vi "Vision Processing Dashboard.vi"() -> (0 "Particle Measurements (Pixels)":dbl[][](array[numeric]))   [LabVIEW 2012]
doc: "<B>Vision Processing Dashboard</B> is a modified FRC Dashboard project that includes vision processing built into the dashboard. The dashboard takes in an image from the camera on the robot and searches for objects within the specified RGB ranges. The image and the image with the threshold are shown in the Camera Image Tab. The ranges are controlled from the Operation tab. The dashboard is set up to display the center of mass in X and Y pixels as well as the area in pixels of any objects that are located."
uses:
  <vilib>/Rock Robotics/WPI/Camera/WPI_CameraImageSize.ctl
  <vilib>/event_ctls.llb/eventvkey.ctl
  <vilib>/Utility/config.llb/Read Key (String).vi
  <vilib>/Utility/config.llb/Read Key (I32).vi
  <vilib>/Analysis/Matrix/Numeric/Conversions/Matrix To Array - RM.vi
  <vilib>/Utility/config.llb/NI_LVConfig.lvlib
  <vilib>/vision/NI_Vision_Development_Module.lvlib
  <vilib>/Analysis/Matrix/NI_Matrix.lvlib
panel:
  out "Battery Value":dbl(slide) scale=0.0..14.0 scale format="%#_2e"
  out "Battery":sgl(graph)
  out "Robot IP":string
  in  "Viewer":T1(tab)
  in  "Enable":bool
  in  "DB Camera Config":bool
  out "Image Error Message":string="Timeout in Camera Communications"
  in  "Camera Address":string="192.168.0.90"
  out "Originial":T2(plugin-control)
  out "Threshold":T2(plugin-control)
  in  "Image Size":T3=enum."320x240"
  out "Buttons 1":cluster{"1":bool, "2":bool, "3":bool}
  out "Kinect 1":cluster{"X":dbl, "Y":dbl, "Z":dbl} {"X" scale=1.0..-1.0; "Y" scale=1.0..-1.0; "Z" scale=1.0..-1.0}
  out "Buttons 2":cluster{"1":bool, "2":bool, "3":bool}
  out "Kinect 2":cluster{"X":dbl, "Y":dbl, "Z":dbl} {"X" scale=1.0..-1.0; "Y" scale=1.0..-1.0; "Z" scale=1.0..-1.0}
  out "Version":string
  out "Skeleton Picture":picture
  out "Players":i8
  out "Tree":string(tree)
  out "Mode":T4(ring)=enum."Auto Disabled"
  out "Camera IP":string
  out "JS1 Z":dbl(slide) scale=-1.0..1.0 scale format="%#_2e"
  out "JS2 Z":dbl(slide) scale=-1.0..1.0 scale format="%#_2e"
  out "Joystick 1":cluster{"X":dbl, "Y":dbl}[](graph)
  out "Joystick 2":cluster{"X":dbl, "Y":dbl}[](graph)
  out "JS Buttons 1":T5
  out "JS Buttons 2":T5
  out "MotorSlide4":dbl(slide) scale=-1.0..1.0 scale format="%#_2e"
  out "MotorSlide3":dbl(slide) scale=-1.0..1.0 scale format="%#_2e"
  out "MotorSlide2":dbl(slide) scale=-1.0..1.0 scale format="%#_2e"
  in  "MotorName3":string="Front Left"
  in  "MotorName4":string="Front Right"
  in  "MotorName1":string="Rear Left"
  in  "MotorName2":string="Rear Right"
  out "MotorChart4":dbl(graph)
  out "MotorChart3":dbl(graph)
  out "MotorChart2":dbl(graph)
  out "MotorSlide1":dbl(slide) scale=-1.0..1.0 scale format="%#_2e"
  out "MotorChart1":dbl(graph)
  in  "Dashboard Tab":enum32{"Operation", "Test", "Checklist"}(tab)
  in  "Red Range":cluster{"Lower value":dbl, "Upper Value":dbl}
  in  "Green Range":cluster{"Lower value":i32, "Upper Value":i32}
  in  "Blue Range":cluster{"Lower value":dbl, "Upper Value":dbl}
  in  "Slider":dbl(slide) scale=0.0..100.0 scale format="%#_3g"
  in  "On/Off":bool caption="Solenoid"
  in  "Test Name":u16(ring) items=["Select the test to run...", "Example Test", "-------------------------------", "List of tests is built in robot code.", "Replace with your own automated tests."]
  in  "Test Tree":string(tree)
  in  "Motor":cluster{"Value":dbl, "Enable":bool} {"Value" scale=-1.0..1.0 scale format="%#_3g"}
  out "Progress":T6 {"Test Progress" scale=0.0..100.0}
  in  "Rev/Fwd":cluster{"Forward":bool, "Reverse":bool}
  in  "Ring":u16(ring) items=["Auto", "Fixed indoor", "Fixed outdoor 1", "Fixed outdoor 2", "Fixed fluorescent 1", "Fixed fluorescent 2", "Hold current"]
  in  "Listbox":i32(listbox)
  # "Robot IP:"
  # "Drive & Motors"
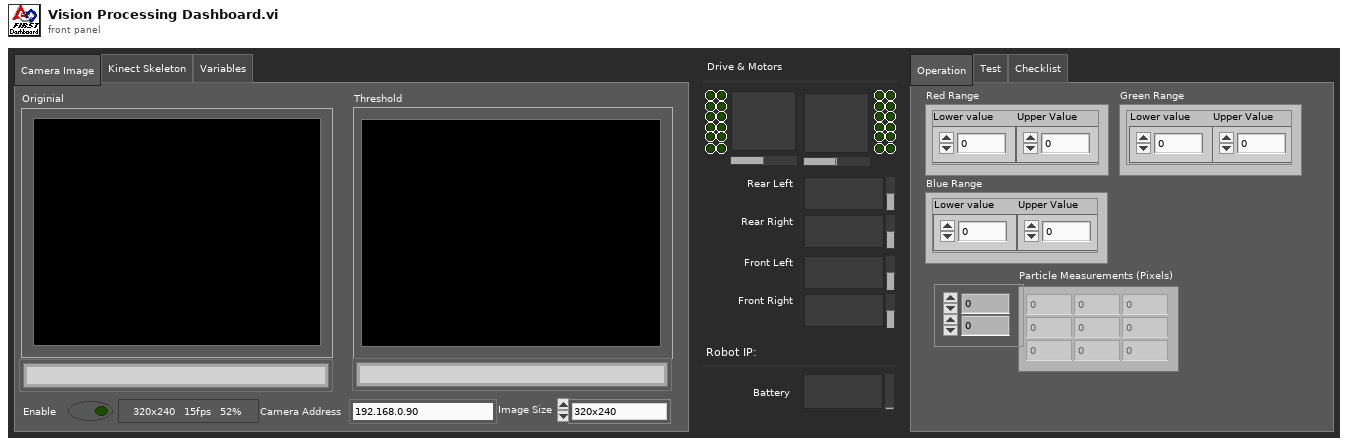
[diagram p1: front panel]
types:
  T1 = enum32{"Camera Image", "Kinect Skeleton", "Variables"}
  T2 = typedef "IMAQ Image.ctl" = refnum<image>
  T3 = typedef "WPI_CameraImageSize.ctl" = enum16{"640x480", "320x240", "160x120"}
  T4 = enum8{"Tele-Op Disabled", "Tele-Op Enabled", "Auto Disabled", "Auto Enabled", "Test Disabled", "Test Enabled", ""}
  T5 = cluster{bool, bool, bool, bool, bool, bool, bool, bool, bool, bool, bool, bool}
  T6 = cluster{"Test Progress":u8, "Test Progress Text":string}
  T7 = typedef "Image Type" = u32
  T8 = typedef "WPI_CameraDevRef.ctl" = cluster{"Camera Address":string, "CameraStatus":errorcluster, "Acquire Image Notifier":refnum<notifier>}
  T9 = typedef "LVBoundsTypeDef.ctl" = cluster{"Width":u32, "Height":u32}
  T10 = typedef "SkeletonTrackState.ctl" = enum32{"NotTracked", "PositionOnly", "Tracked"}
  T11 = cluster{"TrackingState":u8[], "Position":cluster{"x":sgl, "y":sgl, "z":sgl}, cluster{"x":sgl, "y":sgl, "z":sgl, sgl}[], "TrackState":T10}
  T12 = cluster{cluster{"ScaledToPercentRange":dbl, "ScaledToPercentRange":dbl, "ScaledToPercentRange":dbl}, cluster{bool, bool, bool}}[]
  T13 = cluster{cluster{"ScaledToPercentRange":dbl, "ScaledToPercentRange":dbl, "ScaledToPercentRange":dbl}, cluster{bool, bool, bool}}
  T14 = cluster{"ScaledToPercentRange":dbl, "ScaledToPercentRange":dbl, "ScaledToPercentRange":dbl}
  T15 = typedef "LVRectTypeDef.ctl" = cluster{"Left":i16, "Top":i16, "Right":i16, "Bottom":i16}
  T16 = typedef "Particle Parameters" = i32
  T17 = cluster{"[0]":dbl, "[1]":dbl, "[2]":dbl, "[3]":dbl, "[4]":dbl, "[5]":dbl, "[6]":dbl, "[7]":dbl, "[8]":dbl}
  T18 = cluster{"Competition mode":bool, "Robot Link":bool, "Autonomous":bool, "Enabled":bool, "E-Stop":bool, "Simulated":bool, "TestMode":bool, "Docked Window":bool}
  T19 = cluster{"Boolean Array[0]":bool, "Boolean Array[1]":bool, "Boolean Array[2]":bool, "Boolean Array[3]":bool, "Boolean Array[4]":bool, "Boolean Array[5]":bool, "Boolean Array[6]":bool, "Boolean Array[7]":bool, "Boolean Array[8]":bool, "Boolean Array[9]":bool, "Boolean Array[10]":bool, "Boolean Array[11]":bool}
  T20 = typedef "NI_LVConfig.lvlib/Config Data RefNum.ctl" = refnum<k1>
  T21 = typedef "eventvkey.ctl" = enum16{"ASCII", "Enter", "Return", "Shift", "Ctrl", "Alt", "Cmd", "Opt", "Caps", "NumLock", "Clear", "Break", "Up", "Down", "Left", "Right", "Insert", "Delete", "Home", "End", "PageUp", "PageDown", "Escape", "Help", "Pause", "ScrollLock", "F1", "F2", "F3", "F4", "F5", "F6", "F7", "F8", "F9", "F10", "F11", "F12", "F13", "F14", "F15", "F16", "F17", "F18", "F19", "F20", "F21", "F22", "F23", "F24", "Play", "VolumeUp", "VolumeDown", "Mute", "Two Byte Char"}
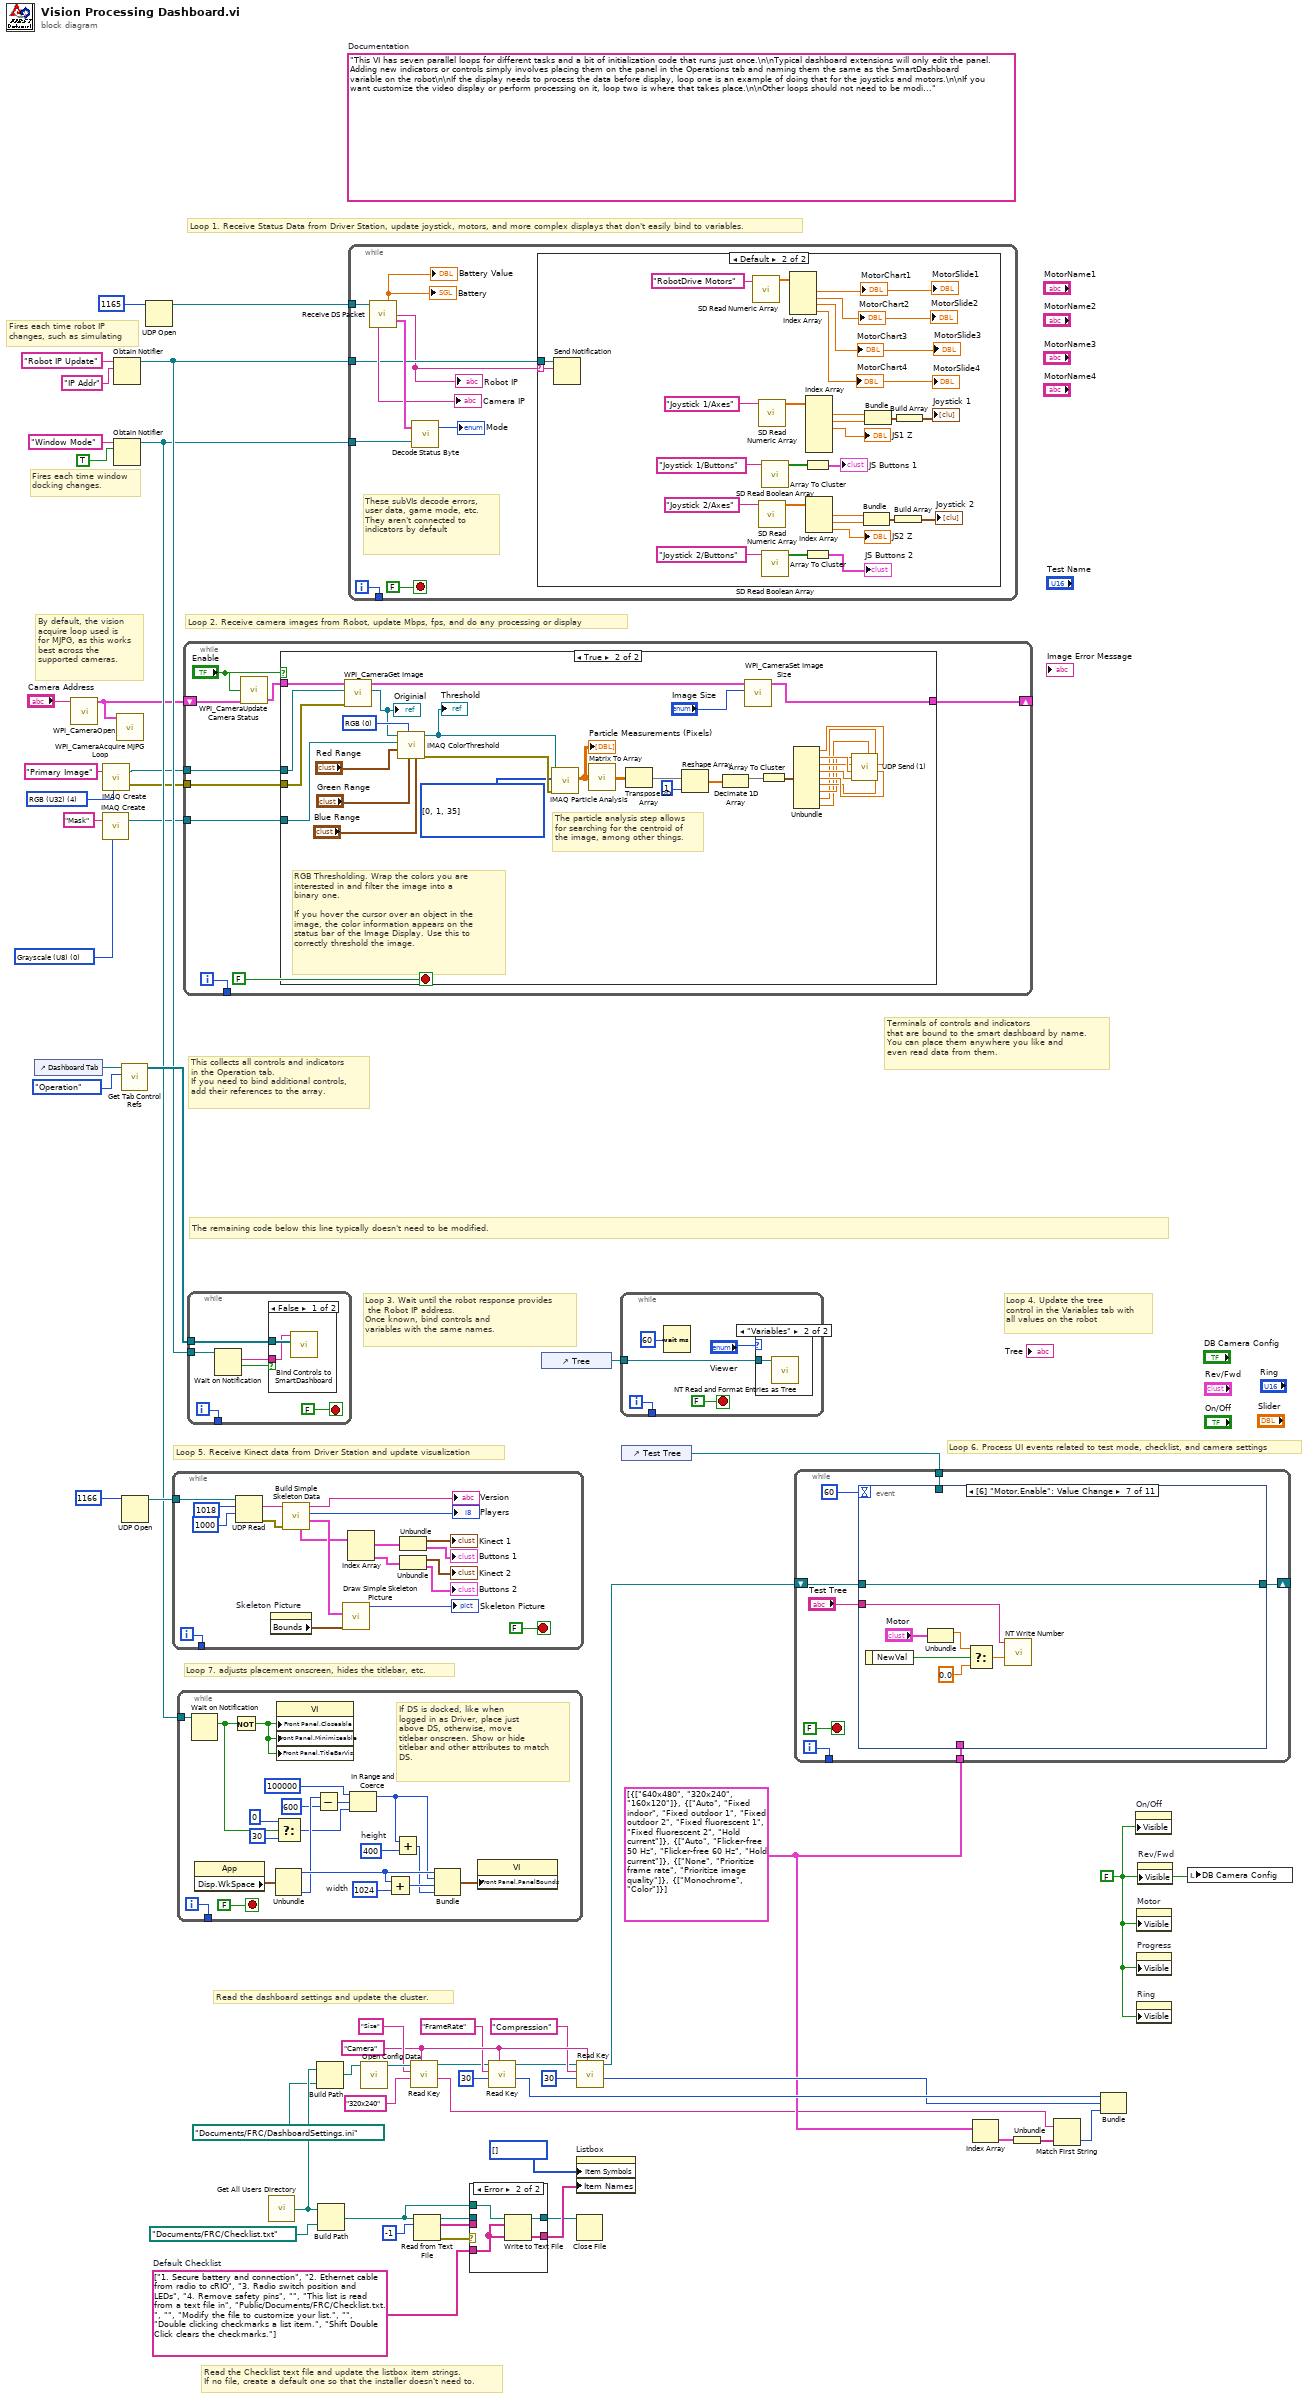
[diagram p0: block diagram]
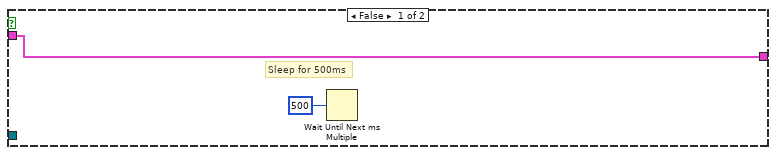
[diagram p3: hidden frame]
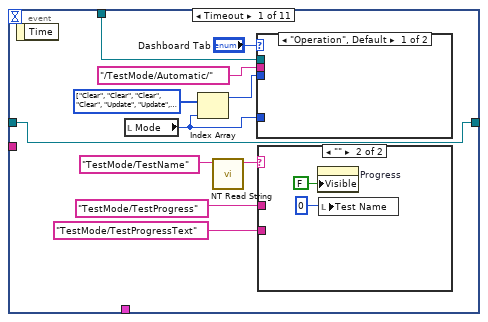
[diagram p5: hidden frame]
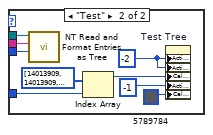
[diagram p6: hidden frame]
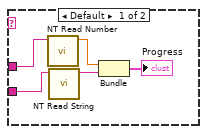
[diagram p7: hidden frame]
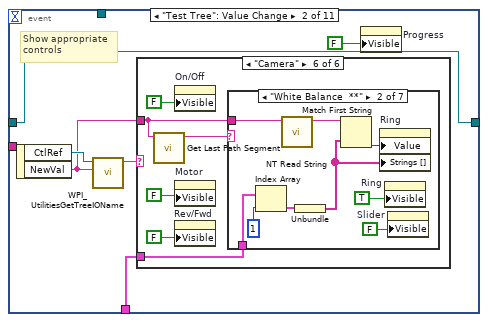
[diagram p8: hidden frame]
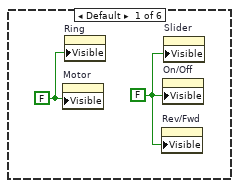
[diagram p9: hidden frame]
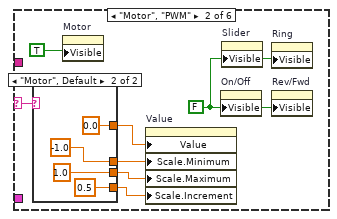
[diagram p10: hidden frame]
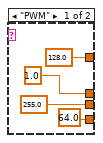
[diagram p11: hidden frame]
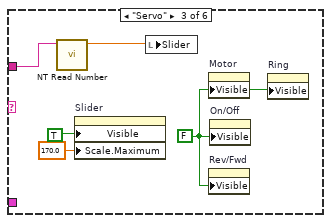
[diagram p12: hidden frame]
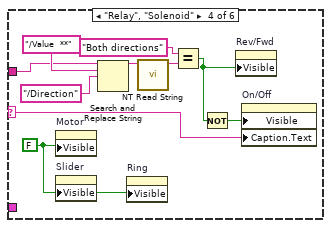
[diagram p13: hidden frame]
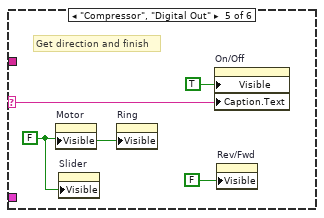
[diagram p14: hidden frame]
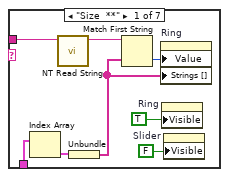
[diagram p15: hidden frame]
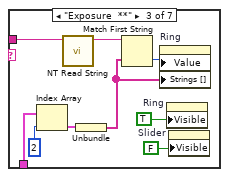
[diagram p16: hidden frame]
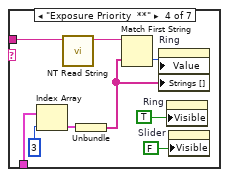
[diagram p17: hidden frame]
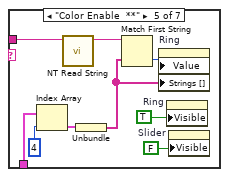
[diagram p18: hidden frame]
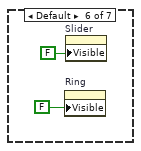
[diagram p19: hidden frame]
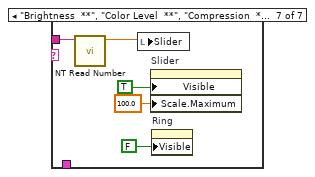
[diagram p20: hidden frame]
diagram:
  w7 = T7 0 items=["Grayscale (U8)", "Grayscale (I16)", "Grayscale (SGL)", "Complex (CSG)", "RGB (U32)", "HSL (U32)", "RGB (U64)", "Grayscale (U16)"] ("Image Type")
  w9 = T7 4 items=["Grayscale (U8)", "Grayscale (I16)", "Grayscale (SGL)", "Complex (CSG)", "RGB (U32)", "HSL (U32)", "RGB (U64)"] ("Image Type")
  w29 = "Camera"
  w21 = cluster{string[]}[] [{["640x480", "320x240", "160x120"]}, {["Auto", "Fixed indoor", "Fixed outdoor 1", "Fixed outdoor 2", "Fixed fluorescent 1", "Fixed fluorescent 2", "Hold current"]}, {["Auto", "Flicker-free 50 Hz", "Flicker-free 60 Hz", "Hold current"]}, {["None", "Prioritize frame rate", "Prioritize image quality"]}, {["Monochrome", "Color"]}]
  w37 = string[] ["1. Secure battery and connection", "2. Ethernet cable from radio to cRIO", "3. Radio switch position and LEDs", "4. Remove safety pins", "", "This list is read from a text file in", "Public/Documents/FRC/Checklist.txt.", "", "Modify the file to customize your list.", "", "Double clicking checkmarks a list item.", "Shift Double Click clears the checkmarks."]  # Default Checklist
  w35 = FALSE ("Visible")
  (unwired) "This VI has seven parallel loops for different tasks and a bit of initialization code that runs just once.\n\nTypical dashboard extensions will only edit the panel. Adding new indicators or controls simply involves placing them on the panel in the Operations tab and naming them the same as the SmartDashboard variable on the robot\n\nIf the display needs to process the data before display, loop one is an example of doing that for the joysticks and motors.\n\nIf you want customize the video display or perform processing on it, loop two is where that takes place.\n\nOther loops should not need to be modified. They are pretty standard, and document the task they perform."  # Documentation
  # "By default, the vision\nacquire loop used is\nfor MJPG, as this works\nbest across the\nsupported cameras."
  # "Fires each time robot IP\nchanges, such as simulating"
  # "Fires each time window\ndocking changes."
  # "Read the Checklist text file and update the listbox item strings.\nIf no file, create a default one so that the installer doesn't need to."
  # "This collects all controls and indicators\nin the Operation tab.\nIf you need to bind additional controls,\nadd their references to the array."
  # "The remaining code below this line typically doesn't need to be modified."
  # "Loop 6. Process UI events related to test mode, checklist, and camera settings"
  # "Read the dashboard settings and update the cluster."
  # "Terminals of controls and indicators\nthat are bound to the smart dashboard by name.\nYou can place them anywhere you like and\neven read data from them."
  # "Loop 4. Update the tree\ncontrol in the Variables tab with\nall values on the robot"
  # "Loop 3. Wait until the robot response provides\n the Robot IP address.\nOnce known, bind controls and\nvariables with the same names."
  # "Loop 5. Receive Kinect data from Driver Station and update visualization"
  # "Loop 7. adjusts placement onscreen, hides the titlebar, etc."
  # "Loop 1. Receive Status Data from Driver Station, update joystick, motors, and more complex displays that don't easily bind to variables."
  # "Loop 2. Receive camera images from Robot, update Mbps, fps, and do any processing or display"
  n1 = control-ref of="Dashboard Tab"() -> (w51:refnum<vi>)
  n2 = call <vilib>:"WPI_CameraOpen.vi"("Camera Address"="Camera Address") -> ("CameraDevRef"=w2:T8)  [unwired: 9 in, 1 out]
  n3 = call "IMAQ Create"("Image Name"="Mask", "Image Type"=w7) -> ("New Image"=w1:T2)  [unwired: 2 in, 2 out]
  n4 = call "IMAQ Create"("Image Name"="Primary Image", "Image Type"=w9) -> ("New Image"=w5:T2, "error out"=w4:errorcluster)  [unwired: 2 in, 1 out]
  n5 = Obtain Notifier(name (unnamed)="Robot IP Update", notification data type="IP Addr" ("name (unnamed)")) -> (notifier out=w48:refnum<notifier>)  [unwired: 2 in, 2 out]
  n6 = Obtain Notifier(name (unnamed)="Window Mode", notification data type=TRUE) -> (notifier out=w41:refnum<notifier>)  [unwired: 2 in, 2 out]
  n7 = call <vilib>:"WPI_CameraAcquire MJPG Loop.vi"("CameraDevRef"=w2) -> ()  [unwired: 11 in]
  n8 = call <vilib>:"Get Tab Control Refs.vi"("Page Index"=enum32{"Operation", "Test"}."Operation" ("Dashboard Tab"), "TabControl in"=w51) -> ("ControlsOnPage"=w52:refnum<vi>[])  [unwired: 9 in]
  n9 = UDP Open(11:u16 1166 ("port")) -> (port=w53:refnum<k16>)  [unwired: 2 in, 4 out]
  n10 = UDP Open(11:u16 1165 ("port")) -> (port=w55:refnum<k16>)  [unwired: 2 in, 4 out]
  n11 = while {
    tunnel: w53 -> [w73]
    tunnel: [w58] -> _
    i -> [w58]
    stop <- FALSE stop-if-true
    n12 = UDP Read(connection ID=w73, max size (548)=1018 ("bytes to read"), timeout ms (25000)=1000) -> (data out=w67:string, error out=w57:errorcluster)  [unwired: 1 in, 3 out]
    n13 = property on="Skeleton Picture" class="Pict"() -> ("Bounds"=w69:T9)  [unwired: 2 in, 2 out]
    n14 = call "Build Simple Skeleton Data.vi"("error in (no error)"=w57, "data in"=w67) -> ("Skeleton Data"=w68:T11, "NumPlayers"=→"Players":i8, "Version String"=→"Version":string, "Simple Joystick Info"=w65:T12)  [unwired: 5 in, 1 out]
    n15 = call "Draw Simple Skeleton Picture.vi"("Bounds"=w69, "Simple Skeleton"=w68) -> ("new picture out"=→"Skeleton Picture":picture)  [unwired: 9 in]
    n16 = Index Array(array=w65) -> (element #1=w64:T13, element #2=w63:T13)  [unwired: 2 in]
    n17 = Unbundle(w64) -> (→"Kinect 1":T14, →"Buttons 1":cluster{bool, bool, bool})
    n18 = Unbundle(w63) -> (→"Kinect 2":T14, →"Buttons 2":cluster{bool, bool, bool})
  }
  n19 = while {
    tunnel: w41 -> [w94]
    tunnel: [w92] -> _
    i -> [w92]
    stop <- FALSE stop-if-true
    w84 = 1024  # width
    w87 = 400  # height
    # "If DS is docked, like when\nlogged in as Driver, place just\nabove DS, otherwise, move\ntitlebar onscreen. Show or hide\ntitlebar and other attributes to match\nDS."
    n20 = Wait on Notification(notifier=w94) -> (notification=w79:bool)  [unwired: 3 in, 3 out]
    n21 = property class="App"() -> ("Disp.WkSpace"=w90:T15)  [unwired: 2 in, 2 out]
    n22 = Not(x=w79) -> (.not. x?=w93:bool)
    n23 = Unbundle(w90) -> ("Left"=w88:i16, "Bottom"=w85:i16)  [unwired: 2 out]
    n24 = Select(t=0, s=w79, f=30) -> (s? t:f=w78:i32)
    n25 = property class="VI"("Front Panel.Closeable"=w93, "Front Panel.Minimizeable"=w93, "Front Panel.TitleBarVis"=w93) -> ()  [unwired: 2 in, 2 out]
    n26 = Subtract(x=w85, y=600) -> (x-y=w82:i32)
    n27 = In Range and Coerce(upper limit=100000, x=w82, lower limit=w78) -> (coerced(x)=w76:i32)  [unwired: 1 out]
    n28 = Add(x=w88, y=w84) -> (x+y=w89:i32)
    n29 = Add(x=w76, y=w87) -> (x+y=w86:i32)
    n30 = Bundle("Left"=w88, w76, w89, w86) -> (w91:cluster{"Left":i16, i32, i32, i32})  [unwired: 1 out]
    n31 = property class="VI"("Front Panel.PanelBounds"=w91) -> ()  [unwired: 2 in, 2 out]
  }
  n32 = while {
    tunnel: w5 -> [w100]
    tunnel: w4 -> [w99]
    tunnel: [w103] -> _
    shift-right: [w97] -> _
    shift-left: w2 -> [w101]
    tunnel: w1 -> [w96]
    i -> [w103]
    stop <- FALSE stop-if-true
    n33 = call <vilib>:"WPI_CameraUpdate Camera Status.vi"("CameraDevRef In"=w101, "Enable Vision"="Enable") -> ("CameraDevRef Out"=w98:T8)  [unwired: 3 in]
    n34 = case shown="True" "Enable" {
      tunnel: w100 -> [_ w137]
      tunnel: w99 -> [_ w136]
      tunnel: w98 -> [w105 w135]
      tunnel: [w105 w126] -> w97
      tunnel: w96 -> [_ w132]
      frame False {
        # "Sleep for 500ms"
        n35 = Wait Until Next ms Multiple(millisecond multiple=u32 500) -> ()  [unwired: 1 out]
      }
      frame True {
        w123 = T16[] [0, 1, 35] items=["Center of Mass X", "Center of Mass Y", "First Pixel X", "First Pixel Y", "Bounding Rect Left", "Bounding Rect Top", "Bounding Rect Right", "Bounding Rect Bottom", "Max Feret Diameter Start X", "Max Feret Diameter Start Y", "Max Feret Diameter End X", "Max Feret Diameter End Y", "Max Horiz. Segment Length Left", "Max Horiz. Segment Length Right", "Max Horiz. Segment Length Row", "-", "Bounding Rect Width", "Bounding Rect Height", "Bounding Rect Diagonal", "Perimeter", "Convex Hull Perimeter", "Holes' Perimeter", "Max Feret Diameter", "Equivalent Ellipse Major Axis", "Equivalent Ellipse Minor Axis", "Equivalent Ellipse Minor Axis (Feret)", "Equivalent Rect Long Side", "Equivalent Rect Short Side", "Equivalent Rect Diagonal", "Equivalent Rect Short Side (Feret)", "Average Horiz. Segment Length", "Average Vert. Segment Length", "Hydraulic Radius", "Waddel Disk Diameter", "-", "Area", "Holes' Area", "Particle & Holes' Area", "Convex Hull Area", "Image Area", "-", "Number of Holes", "Number of Horiz. Segments", "Number of Vert. Segments", "-", "Orientation", "Max Feret Diameter Orientation", "-", "% Area/Image Area", "% Area/(Particle & Holes' Area)", "Ratio of Equivalent Ellipse Axes", "Ratio of Equivalent Rect Sides", "-", "Elongation Factor", "Compactness Factor", "Heywood Circularity Factor", "Type Factor", "-", "Sum X", "Sum Y", "Sum XX", "Sum XY", "Sum YY", "Sum XXX", "Sum XXY", "Sum XYY", "Sum YYY", "-", "Moment of Inertia XX", "Moment of Inertia XY", "Moment of Inertia YY", "Moment of Inertia XXX", "Moment of Inertia XXY", "Moment of Inertia XYY", "Moment of Inertia YYY", "Norm. Moment of Inertia XX", "Norm. Moment of Inertia XY", "Norm. Moment of Inertia YY", "Norm. Moment of Inertia XXX", "Norm. Moment of Inertia XXY", "Norm. Moment of Inertia XYY", "Norm. Moment of Inertia YYY", "Hu Moment 1", "Hu Moment 2", "Hu Moment 3", "Hu Moment 4", "Hu Moment 5", "Hu Moment 6", "Hu Moment 7"] ("Pixel Measurements")
        w134 = u16 0 items=["RGB", "HSL", "HSV", "HSI"] ("Color Mode")
        # "The particle analysis step allows\nfor searching for the centroid of\nthe image, among other things."
        # "RGB Thresholding. Wrap the colors you are\ninterested in and filter the image into a\nbinary one.\n\nIf you hover the cursor over an object in the\nimage, the color information appears on the\nstatus bar of the Image Display. Use this to\ncorrectly threshold the image."
        n36 = call <vilib>:"WPI_CameraGet Image.vi"("error in (no error)"=w136, "Image"=w137, "CameraDevRef"=w135) -> ("Image Out"=w133:T2, "CameraDevRef Out"=w127:T8)  [unwired: 7 out]
        "Originial" <- w133
        n37 = call "IMAQ ColorThreshold"("Blue or Luma or Val or Inten Range"="Blue Range", "Green or Sat Range"="Green Range", "Color Mode"=w134, "Red or Hue Range"="Red Range", "Image Dst"=w132, "Image Src"=w133) -> ("error out"=w129:errorcluster, "Image Dst Out"=w130:T2)  [unwired: 2 in, 2 out]
        "Threshold" <- w130
        n38 = call "IMAQ Particle Analysis"("error in (no error)"=w129, "Pixel Measurements"=w123, "Image"=w130) -> ("Particle Measurements (Pixels)"=w108:dbl[][])  [unwired: 2 in, 6 out]
        "Particle Measurements (Pixels)" <- w108
        n39 = call-poly <vilib>:"Matrix To Array.vi"("Real Matrix"=w108) -> ("Real 2D Array"=w122:dbl[][])
        n40 = Transpose 2D Array(2D array=w122) -> (transposed array=w121:dbl[][])
        n41 = Reshape Array(w121, 1 ("dimension size")) -> (w119:dbl[])
        n42 = Decimate 1D Array(w119) -> (w118:dbl[])  [unwired: 1 out]
        n43 = call <vilib>:"WPI_CameraSet Image Size.vi"("Image Size"="Image Size", "CameraDevRef"=w127) -> ("CameraDevRef Out"=w126:T8)  [unwired: 8 in, 1 out]
        n44 = Array To Cluster(array=w118) -> (cluster=w117:T17)
        n45 = Unbundle(w117) -> ("[0]"=w116:dbl, "[1]"=w115:dbl, "[2]"=w114:dbl, "[3]"=w113:dbl, "[4]"=w112:dbl, "[5]"=w111:dbl, "[6]"=w110:dbl, "[7]"=w109:dbl, "[8]"=w107:dbl)
        n46 = call "UDP Send (1).vi"("Numeric 7"=w110, "Numeric 3"=w114, "Numeric 2"=w115, "Numeric 4"=w113, "Numeric 9"=w107, "Numeric 8"=w109, "Numeric"=w116, "Numeric 5"=w112, "Numeric 6"=w111) -> ()
      }
    }
  }
  n47 = while {
    tunnel: w52 -> [w143]
    tunnel: w48 -> [w140]
    tunnel: [w138] -> _
    i -> [w138]
    stop <- FALSE stop-if-true
    n48 = Wait on Notification(notifier=w140) -> (notification=w139:string, timed out?=w141:bool)  [unwired: 3 in, 2 out]
    n49 = case shown="False" w141 {
      tunnel: w143 -> [w145 _]
      tunnel: w139 -> [w144 _]
      frame False {
        n50 = call <vilib>:"Bind Controls to SmartDashboard.vi"("Bound Control Refs"=w145, "Server IP Address"=w144) -> ()  [unwired: 10 in]
      }
      frame True {
      }
    }
  }
  n51 = call "Get All Users Directory.vi"() -> ("All User Path"=w34:path)
  n52 = Build Path(base path=w34, name or relative path=path "Documents/FRC/DashboardSettings.ini") -> (appended path=w33:path)
  n53 = Build Path(base path=w34, name or relative path=path "Documents/FRC/Checklist.txt") -> (appended path=w38:path)
  n54 = while {
    tunnel: w55 -> [w153]
    tunnel: w48 -> [w147]
    tunnel: w41 -> [w151]
    tunnel: [w148] -> _
    i -> [w148]
    stop <- FALSE stop-if-true
    # "These subVIs decode errors, user data, game mode, etc.\nThey aren't connected to indicators by default"
    n55 = call "Receive DS Packet.vi"("Recv Socket"=w153) -> ("Battery"=→"Battery" →"Battery Value":sgl, "Robot IP Address"=w146:string, "Status"=w154:T18, "Camera IP Address"=→"Camera IP":string)  [unwired: 1 in, 10 out]
    "Robot IP" <- w146
    n56 = call "Decode Status Byte.vi"("Window Mode Notifier"=w151, "Status"=w154) -> ("Mode"=→"Mode":T4)  [unwired: 1 out]
    n57 = case shown="Default" w146 {
      selector: w146 -> [_ w156]
      tunnel: w147 -> [_ w157]
      frame "0.0.0.0" {
        # "Robot not responding, don't poll the variables"
      }
      frame Default {
        n58 = Send Notification(notification=w156, notifier=w157) -> ()  [unwired: 1 in, 2 out]
        n59 = call <vilib>:"SD Read Numeric Array.vi"("Name"="RobotDrive Motors") -> ("Numeric Array"=w180:dbl[])  [unwired: 8 in, 2 out]
        n60 = call <vilib>:"SD Read Numeric Array.vi"("Name"="Joystick 1/Axes") -> ("Numeric Array"=w173:dbl[])  [unwired: 8 in, 2 out]
        n61 = call <vilib>:"SD Read Numeric Array.vi"("Name"="Joystick 2/Axes") -> ("Numeric Array"=w167:dbl[])  [unwired: 8 in, 2 out]
        n62 = call <vilib>:"SD Read Boolean Array.vi"("Name"="Joystick 1/Buttons") -> ("Boolean Array"=w175:bool[])  [unwired: 8 in, 2 out]
        n63 = call <vilib>:"SD Read Boolean Array.vi"("Name"="Joystick 2/Buttons") -> ("Boolean Array"=w166:bool[])  [unwired: 8 in, 2 out]
        n64 = Index Array(array=w180) -> (element #1=→"MotorChart1" →"MotorSlide1":dbl, element #2=→"MotorSlide2" →"MotorChart2":dbl, element #3=→"MotorChart3" →"MotorSlide3":dbl, element #4=→"MotorChart4" →"MotorSlide4":dbl)  [unwired: 4 in]
        n65 = Array To Cluster(array=w175) -> (cluster=→"JS Buttons 1":T19)
        n66 = Array To Cluster(array=w166) -> (cluster=→"JS Buttons 2":T19)
        n67 = Index Array(array=w173) -> (element #1=w170:dbl, element #2=w171:dbl, element #3=→"JS1 Z":dbl)  [unwired: 6 in, 3 out]
        n68 = Index Array(array=w167) -> (element #1=w162:dbl, element #2=w161:dbl, element #3=→"JS2 Z":dbl)  [unwired: 3 in]
        n69 = Bundle("Numeric"=w162, "Numeric"=w161) -> (w163:cluster{"Numeric":dbl, "Numeric":dbl})  [unwired: 1 in]
        n70 = Bundle("Numeric"=w170, "Numeric"=w171) -> (w169:cluster{"Numeric":dbl, "Numeric":dbl})  [unwired: 1 in]
        n71 = Build Array(w163) -> (→"Joystick 2":cluster{"Numeric":dbl, "Numeric":dbl}[])
        n72 = Build Array(w169) -> (→"Joystick 1":cluster{"Numeric":dbl, "Numeric":dbl}[])
      }
    }
  }
  n73 = call <vilib>:"Open Config Data.vi"("configuration file path"=w33) -> ("refnum"=w32:T20)  [unwired: 8 in, 2 out]
  n74 = call-poly <vilib>:"Read Key.vi"("section"=w29, "default value"="320x240", "key"="Size", "refnum"=w32) -> ("value"=w19:string, "refnum out"=w14:T20)  [unwired: 2 in, 4 out]
  n75 = Read from Text File(file (use dialog)=w38, count=-1 ("timeout ms (25000)")) -> (refnum out=w16:refnum<file>, text=w39:string[], error out=w40:errorcluster)  [unwired: 2 in, 1 out]
  n76 = case shown="Error" w40 {
    tunnel: w39 -> [w185 _]
    tunnel: [w185 w187] -> w36
    tunnel: w37 -> [_ w187]
    tunnel: w38 -> [_ w188]
    tunnel: [w184 w186] -> w15
    tunnel: w16 -> [w184 _]
    frame No Error {
    }
    frame Error {
      n77 = Write to Text File(file (use dialog)=w188, text=w187) -> (refnum out=w186:refnum<file>)  [unwired: 2 in, 2 out]
    }
  }
  n78 = call-poly <vilib>:"Read Key.vi"("section"=w29, "default value"=30, "key"="FrameRate", "refnum"=w14) -> ("value"=w24:i32, "refnum out"=w13:T20)  [unwired: 1 in, 5 out]
  n79 = control-ref of="Tree"() -> (w11:refnum<vi>)
  n80 = property on="Listbox" class="LstBox (strict)"("Item Symbols"=i32[] [], "Item Names"=w36) -> ()  [unwired: 2 in, 2 out]
  n81 = Close File(refnum=w15) -> ()  [unwired: 1 in, 2 out]
  n82 = call-poly <vilib>:"Read Key.vi"("section"=w29, "default value"=30, "key"="Compression", "refnum"=w13) -> ("value"=w23:i32, "refnum out"=w12:T20)  [unwired: 1 in, 5 out]
  n83 = while {
    tunnel: [w190] -> _
    tunnel: w11 -> [w189]
    i -> [w190]
    stop <- FALSE stop-if-true
    n84 = Wait (ms)(milliseconds to wait=u32 60) -> ()  [unwired: 1 out]
    n85 = case shown="\"Variables\"" "Viewer" {
      tunnel: w189 -> [_ w194]
      frame Default {
      }
      frame "Variables" {
        n86 = call <vilib>:"NT Read and Format Entries as Tree.vi"("Tree Refnum"=w194) -> ()  [unwired: 9 in, 2 out]
      }
    }
  }
  n87 = control-ref of="Test Tree"() -> (w10:refnum<vi>)
  n88 = while {
    tunnel: w21 -> [w199]
    shift-right: [w198] -> _
    shift-left: w12 -> [w197]
    tunnel: [w196] -> _
    tunnel: w10 -> [w195]
    i -> [w196]
    stop <- FALSE stop-if-true
    n89 = event shown="[6] \"Motor.Enable\": Value Change" {
      selector: _ -> [_ _ _ _ _ _ _ _ _ _ _]
      dyn-events: _ -> [_ _ _ _ _ _ _ _ _ _ _]
      timeout: u32 60 ("milliseconds to wait") -> [_ _ _ _ _ _ _ _ _ _ _]
      tunnel: w195 -> [w209 _ _ _ _ _ _ _ _ _ _]
      tunnel: "Test Tree" -> [_ _ _ _ _ _ w366 w374 w376 w380 w388]
      tunnel: w199 -> [_ w231 _ _ _ _ _ _ _ _ _]
      tunnel: [w203 w230 _ w333 w341 w353 w365 w372 w375 w379 w387] -> w198
      tunnel: w197 -> [w203 w230 _ w333 w341 w353 w365 w372 w375 w379 w387]
      event Timeout {
        w208 = enum16{"Update", "Clear"}[] [enum."Clear", enum."Clear", enum."Clear", enum."Clear", enum."Update", enum."Update", enum."Clear"] items=["Update", "Clear"]
        n90 = event-data() -> ()  [unwired: 1 in, 1 out]
        n91 = local read "Mode"() -> (w206:T4)
        n92 = Index Array(array=w208, index=w206) -> (element=w207:enum16{"Update", "Clear"})
        n93 = call <vilib>:"NT Read String.vi"("Name"="TestMode/TestName") -> ("String"=w212:string)  [unwired: 9 in, 1 out]
        n94 = case shown="\"Operation\", Default" "Dashboard Tab" {
          tunnel: w209 -> [_ w222]
          tunnel: "/TestMode/Automatic/" ("Name Pattern") -> [_ w221]
          tunnel: w207 -> [_ w220]
          tunnel: w206 -> [_ w218]
          frame "Operation", Default {
          }
          frame "Test" {
            w217 = -2 ("Active Item:Row Number")
            n95 = call <vilib>:"NT Read and Format Entries as Tree.vi"("Operation"=w220, "Name Pattern"=w221, "Tree Refnum"=w222) -> ()  [unwired: 7 in, 2 out]
            n96 = Index Array(array=u32[] [14013909, 14013909, 14013909, 14013909, 14013909, 16777215, 14013909], index=w218) -> (element=w216:u32)
            n97 = property on="Test Tree" class="Tree (strict)"("Active Item Row Number"=w217, "ActiveColNum"=w217, "CellBG"=w216, "Active Item Row Number"=-1 ("Active Item:Row Number"), "CellBG"=u32 5789784 ("Color Box")) -> ()  [unwired: 2 in, 2 out]
          }
        }
        n98 = case shown="\"\"" w212 {
          tunnel: "TestMode/TestProgress" ("Name") -> [w224 _]
          tunnel: "TestMode/TestProgressText" ("Name") -> [w223 _]
          frame Default {
            n99 = call <vilib>:"NT Read Number.vi"("Name"=w224) -> ("Numeric"=w225:dbl)  [unwired: 9 in, 1 out]
            n100 = call <vilib>:"NT Read String.vi"("Name"=w223) -> ("String"=w226:string)  [unwired: 9 in, 1 out]
            n101 = Bundle("Numeric"=w225, "String"=w226) -> (→"Progress":cluster{"Numeric":dbl, "String":string})  [unwired: 1 in]
          }
          frame "" {
            n102 = property on="Progress" class="Clust (strict)"("Visible"=FALSE) -> ()  [unwired: 2 in, 2 out]
            n103 = local write "Test Name"(u16 0) -> ()
          }
        }
      }
      event "Test Tree": Value Change {
        # "Show appropriate\ncontrols"
        n104 = event-data() -> ("CtlRef"=w234:refnum<vi>, "NewVal"=w232:string)  [unwired: 1 in]
        n105 = call <vilib>:"WPI_UtilitiesGetTreeIOName.vi"("NewVal"=w232, "TreeControl in"=w234) -> ("I/O Name"=w235:string)  [unwired: 9 in]
        n106 = case shown="\"Camera\"" w235 {
          selector: w235 -> [_ w242 _ w260 w269 _]
          tunnel: w232 -> [_ _ w257 w259 _ w276]
          tunnel: w231 -> [_ _ _ _ _ w275]
          frame Default {
            w237 = FALSE ("Visible")
            w236 = FALSE ("Visible")
            n107 = property on="Motor" class="Clust (strict)"("Visible"=w236) -> ()  [unwired: 2 in, 2 out]
            n108 = property on="Ring" class="Ring (strict)"("Visible"=w236) -> ()  [unwired: 2 in, 2 out]
            n109 = property on="Rev/Fwd" class="Clust (strict)"("Visible"=w237) -> ()  [unwired: 2 in, 2 out]
            n110 = property on="On/Off" class="Bool (strict)"("Visible"=w237) -> ()  [unwired: 2 in, 2 out]
            n111 = property on="Slider" class="Slide (strict)"("Visible"=w237) -> ()  [unwired: 2 in, 2 out]
          }
          frame "Motor", "PWM" {
            w243 = FALSE ("Visible")
            n112 = case shown="\"Motor\", Default" w242 {
              tunnel: [1.0 ("Value") -1.0 ("Value")] -> w241
              tunnel: [255.0 ("Value") 1.0 ("Value")] -> w240
              tunnel: [128.0 ("Value") 0.0 ("Value")] -> w239
              tunnel: [64.0 ("Value") 0.5 ("Value")] -> w238
              frame "PWM" {
              }
              frame "Motor", Default {
              }
            }
            n113 = property on="Motor" class="Clust (strict)"("Visible"=TRUE) -> ()  [unwired: 2 in, 2 out]
            n114 = property on="Value" class="Slide (strict)"("Value"=w239, "Scale.Minimum"=w241, "Scale.Maximum"=w240, "Scale.Increment"=w238) -> ()  [unwired: 2 in, 2 out]
            n115 = property on="On/Off" class="Bool (strict)"("Visible"=w243) -> ()  [unwired: 2 in, 2 out]
            n116 = property on="Slider" class="Slide (strict)"("Visible"=w243) -> ()  [unwired: 2 in, 2 out]
            n117 = property on="Ring" class="Ring (strict)"("Visible"=w243) -> ()  [unwired: 2 in, 2 out]
            n118 = property on="Rev/Fwd" class="Clust (strict)"("Visible"=w243) -> ()  [unwired: 2 in, 2 out]
          }
          frame "Servo" {
            w255 = FALSE ("Visible")
            n119 = call <vilib>:"NT Read Number.vi"("Name"=w257) -> ("Numeric"=w256:dbl)  [unwired: 9 in, 1 out]
            n120 = property on="Slider" class="Slide (strict)"("Visible"=TRUE, "Scale.Maximum"=170.0 ("Scale.Range:Maximum")) -> ()  [unwired: 2 in, 2 out]
            n121 = local write "Slider"(w256) -> ()
            n122 = property on="Motor" class="Clust (strict)"("Visible"=w255) -> ()  [unwired: 2 in, 2 out]
            n123 = property on="Rev/Fwd" class="Clust (strict)"("Visible"=w255) -> ()  [unwired: 2 in, 2 out]
            n124 = property on="On/Off" class="Bool (strict)"("Visible"=w255) -> ()  [unwired: 2 in, 2 out]
            n125 = property on="Ring" class="Ring (strict)"("Visible"=w255) -> ()  [unwired: 2 in, 2 out]
          }
          frame "Relay", "Solenoid" {
            w258 = FALSE ("Visible")
            n126 = property on="Motor" class="Clust (strict)"("Visible"=w258) -> ()  [unwired: 2 in, 2 out]
            n127 = property on="Slider" class="Slide (strict)"("Visible"=w258) -> ()  [unwired: 2 in, 2 out]
            n128 = Search and Replace String(input string=w259, search string="/Value  **", replace string="/Direction") -> (result string=w265:string)  [unwired: 5 in, 3 out]
            n129 = property on="Ring" class="Ring (strict)"("Visible"=w258) -> ()  [unwired: 2 in, 2 out]
            n130 = call <vilib>:"NT Read String.vi"("Name"=w265) -> ("String"=w263:string)  [unwired: 9 in, 1 out]
            n131 = Equal?(x="Both directions", y=w263) -> (x = y?=w261:bool)
            n132 = Not(x=w261) -> (.not. x?=w262:bool)
            n133 = property on="Rev/Fwd" class="Clust (strict)"("Visible"=w261) -> ()  [unwired: 2 in, 2 out]
            n134 = property on="On/Off" class="Bool (strict)"("Visible"=w262, "Caption.Text"=w260) -> ()  [unwired: 2 in, 2 out]
          }
          frame "Compressor", "Digital Out" {
            w268 = FALSE ("Visible")
            # "Get direction and finish"
            n135 = property on="Motor" class="Clust (strict)"("Visible"=w268) -> ()  [unwired: 2 in, 2 out]
            n136 = property on="Slider" class="Slide (strict)"("Visible"=w268) -> ()  [unwired: 2 in, 2 out]
            n137 = property on="Ring" class="Ring (strict)"("Visible"=w268) -> ()  [unwired: 2 in, 2 out]
            n138 = property on="On/Off" class="Bool (strict)"("Visible"=TRUE, "Caption.Text"=w269) -> ()  [unwired: 2 in, 2 out]
            n139 = property on="Rev/Fwd" class="Clust (strict)"("Visible"=FALSE) -> ()  [unwired: 2 in, 2 out]
          }
          frame "Camera" {
            n140 = call <vilib>:"Get Last Path Segment.vi"("String in"=w276) -> ("String out"=w277:string)  [unwired: 10 in]
            n141 = property on="On/Off" class="Bool (strict)"("Visible"=FALSE) -> ()  [unwired: 2 in, 2 out]
            n142 = property on="Motor" class="Clust (strict)"("Visible"=FALSE) -> ()  [unwired: 2 in, 2 out]
            n143 = property on="Rev/Fwd" class="Clust (strict)"("Visible"=FALSE) -> ()  [unwired: 2 in, 2 out]
            n144 = case shown="\"White Balance  **\"" w277 {
              tunnel: w276 -> [w283 w292 w301 w310 w319 _ w325]
              tunnel: w275 -> [w281 w289 w298 w307 w316 _ _]
              frame "Size  **" {
                n145 = Index Array(array=w281) -> (element=w280:cluster{string[]})  [unwired: 1 in]
                n146 = call <vilib>:"NT Read String.vi"("Name"=w283) -> ("String"=w282:string)  [unwired: 9 in, 1 out]
                n147 = Unbundle(w280) -> (w278:string[])
                n148 = Match First String(2:w278, 3:w282) -> (0:w279:i32)  [unwired: 1 out]
                n149 = property on="Ring" class="Ring (strict)"("Value"=w279, "Strings []"=w278) -> ()  [unwired: 2 in, 2 out]
                n150 = property on="Ring" class="Ring (strict)"("Visible"=TRUE) -> ()  [unwired: 2 in, 2 out]
                n151 = property on="Slider" class="Slide (strict)"("Visible"=FALSE) -> ()  [unwired: 2 in, 2 out]
              }
              frame "White Balance  **" {
                n152 = Index Array(array=w289, index=1) -> (element=w290:cluster{string[]})
                n153 = call <vilib>:"NT Read String.vi"("Name"=w292) -> ("String"=w291:string)  [unwired: 9 in, 1 out]
                n154 = Unbundle(w290) -> (w287:string[])
                n155 = Match First String(2:w287, 3:w291) -> (0:w286:i32)  [unwired: 1 out]
                n156 = property on="Ring" class="Ring (strict)"("Value"=w286, "Strings []"=w287) -> ()  [unwired: 2 in, 2 out]
                n157 = property on="Ring" class="Ring (strict)"("Visible"=TRUE) -> ()  [unwired: 2 in, 2 out]
                n158 = property on="Slider" class="Slide (strict)"("Visible"=FALSE) -> ()  [unwired: 2 in, 2 out]
              }
              frame "Exposure  **" {
                n159 = Index Array(array=w298, index=2) -> (element=w299:cluster{string[]})
                n160 = call <vilib>:"NT Read String.vi"("Name"=w301) -> ("String"=w300:string)  [unwired: 9 in, 1 out]
                n161 = Unbundle(w299) -> (w295:string[])
                n162 = Match First String(2:w295, 3:w300) -> (0:w296:i32)  [unwired: 1 out]
                n163 = property on="Ring" class="Ring (strict)"("Value"=w296, "Strings []"=w295) -> ()  [unwired: 2 in, 2 out]
                n164 = property on="Ring" class="Ring (strict)"("Visible"=TRUE) -> ()  [unwired: 2 in, 2 out]
                n165 = property on="Slider" class="Slide (strict)"("Visible"=FALSE) -> ()  [unwired: 2 in, 2 out]
              }
              frame "Exposure Priority  **" {
                n166 = Index Array(array=w307, index=3) -> (element=w308:cluster{string[]})
                n167 = call <vilib>:"NT Read String.vi"("Name"=w310) -> ("String"=w309:string)  [unwired: 9 in, 1 out]
                n168 = Unbundle(w308) -> (w304:string[])
                n169 = Match First String(2:w304, 3:w309) -> (0:w305:i32)  [unwired: 1 out]
                n170 = property on="Ring" class="Ring (strict)"("Value"=w305, "Strings []"=w304) -> ()  [unwired: 2 in, 2 out]
                n171 = property on="Ring" class="Ring (strict)"("Visible"=TRUE) -> ()  [unwired: 2 in, 2 out]
                n172 = property on="Slider" class="Slide (strict)"("Visible"=FALSE) -> ()  [unwired: 2 in, 2 out]
              }
              frame "Color Enable  **" {
                n173 = Index Array(array=w316, index=4) -> (element=w317:cluster{string[]})
                n174 = call <vilib>:"NT Read String.vi"("Name"=w319) -> ("String"=w318:string)  [unwired: 9 in, 1 out]
                n175 = Unbundle(w317) -> (w313:string[])
                n176 = Match First String(2:w313, 3:w318) -> (0:w314:i32)  [unwired: 1 out]
                n177 = property on="Ring" class="Ring (strict)"("Value"=w314, "Strings []"=w313) -> ()  [unwired: 2 in, 2 out]
                n178 = property on="Ring" class="Ring (strict)"("Visible"=TRUE) -> ()  [unwired: 2 in, 2 out]
                n179 = property on="Slider" class="Slide (strict)"("Visible"=FALSE) -> ()  [unwired: 2 in, 2 out]
              }
              frame Default {
                n180 = property on="Ring" class="Ring (strict)"("Visible"=FALSE) -> ()  [unwired: 2 in, 2 out]
                n181 = property on="Slider" class="Slide (strict)"("Visible"=FALSE) -> ()  [unwired: 2 in, 2 out]
              }
              frame "Brightness  **", "Color Level  **", "Compression  **", "FPS  **", "Sharpness  **" {
                n182 = call <vilib>:"NT Read Number.vi"("Name"=w325) -> ("Numeric"=w324:dbl)  [unwired: 9 in, 1 out]
                n183 = local write "Slider"(w324) -> ()
                n184 = property on="Slider" class="Slide (strict)"("Visible"=TRUE, "Scale.Maximum"=100.0 ("Scale.Range:Maximum")) -> ()  [unwired: 2 in, 2 out]
                n185 = property on="Ring" class="Ring (strict)"("Visible"=FALSE) -> ()  [unwired: 2 in, 2 out]
              }
            }
          }
        }
        n186 = property on="Progress" class="Clust (strict)"("Visible"=FALSE) -> ()  [unwired: 2 in, 2 out]
      }
      event "Test Name": Mouse Enter {
        # "Populate the ring with the list of tests"
        n187 = event-data() -> ()  [unwired: 1 in, 1 out]
        n188 = call <vilib>:"NT Read String Array.vi"("Name"="TestMode/TestList") -> ("String Array"=w332:string[])  [unwired: 9 in, 1 out]
        n189 = Build Array (concatenate)("Select the test to run...", w332) -> (w331:string[])
        n190 = property on="Test Name" class="Ring (strict)"("Strings []"=w331) -> ()  [unwired: 2 in, 2 out]
      }
      event "Test Name": Value Change {
        w334 = FALSE ("Visible")
        # "Tell the robot the test name to run"
        n191 = event-data() -> ("NewVal"=w338:u16)  [unwired: 1 in]
        n192 = property on="Test Name" class="Ring (strict)"() -> ("Strings []"=w339:string[])  [unwired: 2 in, 2 out]
        n193 = local write "Progress"(T6 {"Test Progress"=0, "Test Progress Text"=""} ("Progress")) -> ()
        n194 = Index Array(array=w339, index=w338) -> (element=w337:string)
        n195 = call <vilib>:"NT Write String.vi"("String"=w337, "Name"="TestMode/TestName") -> ()  [unwired: 9 in, 1 out]
        n196 = property on="Progress" class="Clust (strict)"("Visible"=TRUE) -> ()  [unwired: 2 in, 2 out]
        n197 = property on="Motor" class="Clust (strict)"("Visible"=w334) -> ()  [unwired: 2 in, 2 out]
        n198 = property on="Slider" class="Slide (strict)"("Visible"=w334) -> ()  [unwired: 2 in, 2 out]
        n199 = property on="On/Off" class="Bool (strict)"("Visible"=w334) -> ()  [unwired: 2 in, 2 out]
        n200 = property on="Rev/Fwd" class="Clust (strict)"("Visible"=w334) -> ()  [unwired: 2 in, 2 out]
        n201 = property on="Ring" class="Ring (strict)"("Visible"=w334) -> ()  [unwired: 2 in, 2 out]
      }
      event "Listbox": Double Click {
        n202 = event-data() -> ("PlatMods.Shift"=w342:bool, "Row"=w344:i32)  [unwired: 1 in]
        n203 = case shown="False" w342 {
          tunnel: w344 -> [w348 _]
          tunnel: 1 -> [w347 _]
          frame False {
            n204 = property on="Listbox" class="LstBox (strict)"() -> ("Item Symbols"=w346:i32[])  [unwired: 2 in, 2 out]
            n205 = Replace Array Subset(array=w346, new element=w347, index=w348) -> (w345:i32[])
            n206 = property on="Listbox" class="LstBox (strict)"("Item Symbols"=w345) -> ()  [unwired: 2 in, 2 out]
          }
          frame True {
            w349 = 0 ("Top Row")
            n207 = property on="Listbox" class="LstBox (strict)"() -> ("Number of Rows"=w351:u32)  [unwired: 2 in, 2 out]
            n208 = Initialize Array(0, w351) -> (w350:i32[])
            n209 = property on="Listbox" class="LstBox (strict)"("Top Row"=w349, "Value"=w349, "Item Symbols"=w350) -> ()  [unwired: 2 in, 2 out]
          }
        }
      }
      event "Listbox": Key Down {
        n210 = event-data() -> ("VKey"=w355:T21)  [unwired: 1 in]
        n211 = case shown="\"Left\", \"Right\"" w355 {
          selector: w355 -> [w360 _]
          tunnel: eventvkey."Left" ("VKey") -> [w358 _]
          frame "Left", "Right" {
            n212 = Equal?(x=w358, y=w360) -> (x = y?=w359:bool)
            n213 = Select(t=0, s=w359, f=1) -> (s? t:f=w361:i32)
            n214 = property on="Listbox" class="LstBox (strict)"() -> ("Item Symbols"=w364:i32[])  [unwired: 2 in, 2 out]
            n215 = Replace Array Subset(array=w364, new element=w361, index="Listbox") -> (w363:i32[])
            n216 = property on="Listbox" class="LstBox (strict)"("Item Symbols"=w363) -> ()  [unwired: 2 in, 2 out]
          }
          frame Default {
          }
        }
      }
      event "Motor.Enable": Value Change {
        n217 = event-data() -> ("NewVal"=w370:bool)  [unwired: 1 in]
        n218 = Unbundle("Motor") -> ("Value"=w369:dbl)  [unwired: 1 out]
        n219 = Select(t=w369, s=w370, f=0.0) -> (s? t:f=w367:dbl)
        n220 = call <vilib>:"NT Write Number.vi"("Numeric"=w367, "Name"=w366) -> ()  [unwired: 9 in, 1 out]
      }
      event "Slider": Value Change {
        n221 = event-data() -> ("NewVal"=w373:dbl)  [unwired: 1 in]
        n222 = call <vilib>:"NT Write Number.vi"("Numeric"=w373, "Name"=w374) -> ()  [unwired: 9 in, 1 out]
      }
      event "On/Off": Value Change {
        n223 = event-data() -> ("NewVal"=w378:bool)  [unwired: 1 in]
        n224 = Boolean To (0,1)(Boolean=w378) -> (0, 1=w377:i16)
        n225 = call <vilib>:"NT Write Number.vi"("Numeric"=w377, "Name"=w376) -> ()  [unwired: 9 in, 1 out]
      }
      event "Rev/Fwd": Value Change {
        n226 = event-data() -> ("NewVal.Forward"=w386:bool, "NewVal.Reverse"=w385:bool)  [unwired: 1 in]
        n227 = Boolean To (0,1)(Boolean=w386) -> (0, 1=w382:i16)
        n228 = Boolean To (0,1)(Boolean=w385) -> (0, 1=w384:i16)
        n229 = Negate(x=w384) -> (-x=w383:i16)
        n230 = Add(x=w382, y=w383) -> (x+y=w381:i16)
        n231 = call <vilib>:"NT Write Number.vi"("Numeric"=w381, "Name"=w380) -> ()  [unwired: 9 in, 1 out]
      }
      event "Ring": Value Change {
        n232 = event-data() -> ("NewVal"=w390:u16)  [unwired: 1 in]
        n233 = property on="Ring" class="Ring (strict)"() -> ("Strings []"=w391:string[])  [unwired: 2 in, 2 out]
        n234 = Index Array(array=w391, index=w390) -> (element=w389:string)
        n235 = call <vilib>:"NT Write String.vi"("String"=w389, "Name"=w388) -> ()  [unwired: 9 in, 1 out]
      }
    }
  }
  n236 = Index Array(array=w21) -> (element=w22:cluster{string[]})  [unwired: 1 in]
  n237 = Unbundle(w22) -> (w20:string[])
  n238 = Match First String(2:w20, 3:w19) -> (0:w18:i32)  [unwired: 1 out]
  n239 = Bundle("value"=w24, "value"=w23, "index"=w18) -> ()  [unwired: 2 out]
  n240 = property on="On/Off" class="Bool (strict)"("Visible"=w35) -> ()  [unwired: 2 in, 2 out]
  n241 = property on="Motor" class="Clust (strict)"("Visible"=w35) -> ()  [unwired: 2 in, 2 out]
  n242 = property on="Progress" class="Clust (strict)"("Visible"=w35) -> ()  [unwired: 2 in, 2 out]
  n243 = property on="Ring" class="Ring (strict)"("Visible"=w35) -> ()  [unwired: 2 in, 2 out]
  n244 = property on="Rev/Fwd" class="Clust (strict)"("Visible"=w35) -> ()  [unwired: 2 in, 2 out]
  n245 = local write "DB Camera Config"(w35) -> ()
